vi "To String and From String Array Test.vi"() -> ()   [LabVIEW 2015, in "Conditional Jump Tests.lvlib"]
uses:
  Conditional Jump Tests.lvlib
  <vilib>/NI/Tag Bus/tag/Data Type.ctl
  <vilib>/NI/Tag Bus Module Framework/channel/channel classification.ctl
  Config/Conditional Jump Step Config.lvclass
  <vilib>/NI/Tag Bus/tag/tag descriptor.lvclass
  <vilib>/NI/Tag Bus Module Framework/channel/TBM channel.lvclass
panel:
  out "Pass":bool
  out "error out":errorcluster
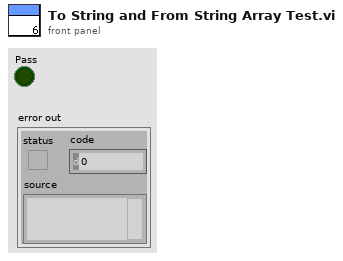
[diagram p1: front panel]
types:
  T1 = typedef "TBM channel.lvclass/channel classification.ctl" = enum16{"input data", "output data", "processing parameter", "processing result"}
  T2 = typedef "tag bus.lvlib/tag descriptor.lvclass/Data Type.ctl" = enum16{"Double", "Single", "I64", "I32", "I16", "I8", "U64", "U32", "U16", "U8", "Boolean", "String", "Array of Double", "Array of Single", "Array of I64", "Array of I32", "Array of I16", "Array of I8", "Array of U64", "Array of U32", "Array of U16", "Array of U8", "Array of Boolean", "Array of String"}
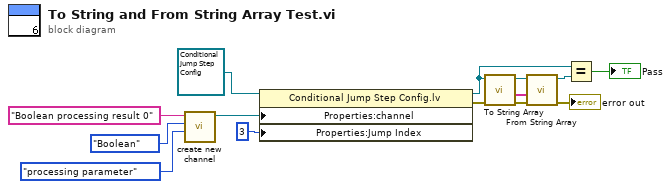
[diagram p0: block diagram]
diagram:
  n1 = call <vilib>:"create new channel.vi"("channel classification"=channel_classification."processing parameter", "data type"=Data_Type."Boolean" ("Data Type"), "channel name"="Boolean processing result 0" ("Jump Tag Name")) -> ("channel"=w11:refnum<class "TBM channel.lvclass">)  [unwired: 8 in]
  n2 = property class="Conditional Jump Step Config.lv"(reference=refnum<class "Conditional Jump Step Config.lvclass"> refnum ("Conditional Jump Step Config.lvclass"), "Properties:channel"=w11, "Properties:Jump Index"=3 ("Jump Index")) -> (reference out=w2:refnum<class "Conditional Jump Step Config.lvclass">, error out=w5:errorcluster)  [unwired: 1 in]
  n3 = call-dynamic "To String Array.vi"("error in (no error)"=w5, "Conditional Jump Step Config in"=w2) -> ("error out"=w6:errorcluster, "Step String Array"=w7:string[], "Conditional Jump Step Config out"=w8:refnum<class "Conditional Jump Step Config.lvclass">)  [unwired: 7 in]
  n4 = call-dynamic "From String Array.vi"("error in (no error)"=w6, "String Array"=w7, "Conditional Jump Step Config in"=w8) -> ("error out"=→"error out":errorcluster, "Conditional Jump Step Config out"=w3:refnum<class "Conditional Jump Step Config.lvclass">)  [unwired: 6 in, 1 out]
  n5 = Equal?(x=w2, y=w3) -> (x = y?=→"Pass":bool)
